vi "Add Error to Display.vi"(8 "error in (no error)":errorcluster, 9 "Update Listbox":bool=TRUE, 10 "error to display":T1 {"Time Stamp" format="%<%x %.3X>T"}, 11 "Error Manager in":refnum<class "Error Manager.lvclass">) -> (0 "error out":errorcluster, 3 "Error Manager out":refnum<class "Error Manager.lvclass">)   [LabVIEW 2026, in "TALOS.lvlib" / "Error Manager.lvlib" / "Error Manager.lvclass"]
uses:
  Error Manager.lvclass
  C:/LabVIEW Code/TALOS/talos/Father of all uServices/Father of all uServices/Father of all uServices.lvclass
  Error Info.ctl
  Error Manager.lvclass/Error Manager.ctl
  Father of all uServices/Father of all uServices/Father of all uServices.lvclass/Father of all uServices.ctl
  Ancestor/Ancestor/Ancestor.lvclass/Ancestor.ctl
  Common GUI v3/Common GUI v3/Error Listbox Msg.ctl
  Common GUI v3/Common GUI v3/Error Listbox Msg Action.ctl
  Guardian/Guardian/Requests.ctl
  Guardian/Guardian Messages/Requests from uServices Msg/Requests from uServices Msg.lvclass/Requests from uServices Msg.ctl
  Support VIs/Substitute Error.vi
  Guardian/Guardian Messages/Requests from uServices Msg/Send Requests from uServices.vi
  Support VIs/Generate Error.vi
  FGV/Error Memory/Get Error Description.vi
  Support VIs/Get PC name.vi
  Ancestor/Ancestor/Read ID.vi
  Support VIs/Get Class Name.vi
  <vilib>/Utility/error.llb/Clear Errors.vi
  FGV/Error Memory/Error Memory Core.vi
  <vilib>/AdvancedString/Delimited String to 1D String Array.vi
  <vilib>/AdvancedString/Delimited String to 1D String Array (string).vi
  Support VIs/Circus Root Path.vi
  FGV/Error Memory/Error Crt Lvl checker.vi
  FGV/Error Memory/Error Memory Core.vi/40c8088d-b597-4017-91af-faa98e00292e.vi
  FGV/Error Memory/Error Memory Core.vi/d4a3ab98-063c-4e44-b43d-fbdcfe6c2be2.vi
  Father of all uServices/Father of all uServices/Father of all uServices.lvclass
  C:/LabVIEW Code/TALOS/builds/Actor Framework PPL/Actor Framework.lvlibp/1abvi3w/vi.lib/ActorFramework/Actor/Actor.lvclass
  Support VIs/Global Memory.vi
  <vilib>/Utility/LVClass/Get LV Class Name.vi
  Support VIs/Is in Packed Library.vi
  Support VIs/TALOS Root path.vi
  Support VIs/Read CSV worksheet.vi
  Support VIs/Global Constants.vi
  <vilib>/Utility/error.llb/General Error Handler.vi
  Support VIs/Error Log.vi
  builds/Actor Framework PPL/Actor Framework.lvlibp/1abvi3w/vi.lib/ActorFramework/Actor/Read Caller Enqueuer.vi
  builds/Actor Framework PPL/Actor Framework.lvlibp/1abvi3w/vi.lib/ActorFramework/Message Enqueuer/Enqueue.vi
  Ancestor/Ancestor/Ancestor.lvclass
  <vilib>/Comparison/Equal/Equal Functor/Equal Functor.lvclass
  Guardian/Guardian Messages/Requests from uServices Msg/Requests from uServices Msg.lvclass
  Guardian/Guardian/Guardian.lvclass
  Common GUI v3/Common GUI v3/Common GUI v3.lvclass
  TALOS.lvlib
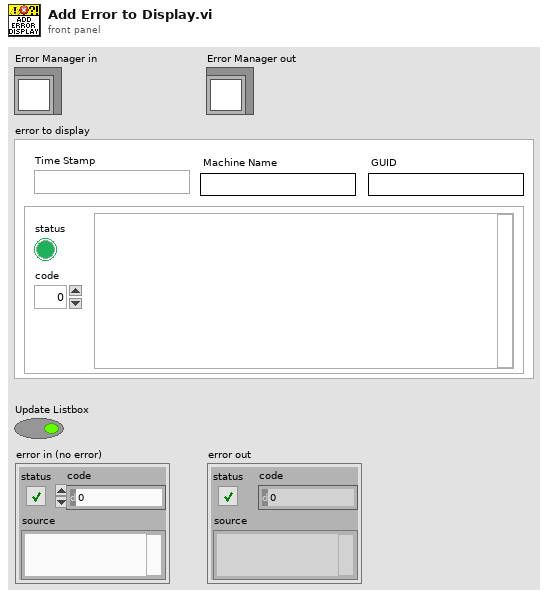
[diagram p1: front panel]
types:
  T1 = typedef "TALOS.lvlib/Error Manager.lvlib/Error Manager.lvclass/Error Info.ctl" = cluster{"error out":errorcluster, "Time Stamp":timestamp, "Machine Name":string, "GUID":string}
  T2 = typedef "TALOS.lvlib/Guardian.lvlib/Guardian.lvclass/Requests.ctl" = enum16{"Ready to Launch", "Start RUN", "Stop RUN", "Update DAQ Params", "Update Error Listbox", "Update Run Status", "Update Kasli Log", "Run Stopped with Errors", "Switch uS View", "Dismiss All Errors"}
  T3 = typedef "TALOS.lvlib/Common GUI v3.lvlib/Common GUI v3.lvclass/Error Listbox Msg Action.ctl" = enum16{"Add", "Remove", "Clear"}
  T4 = typedef "TALOS.lvlib/Common GUI v3.lvlib/Common GUI v3.lvclass/Error Listbox Msg.ctl" = cluster{"Action":T3, "Error Info":T1}
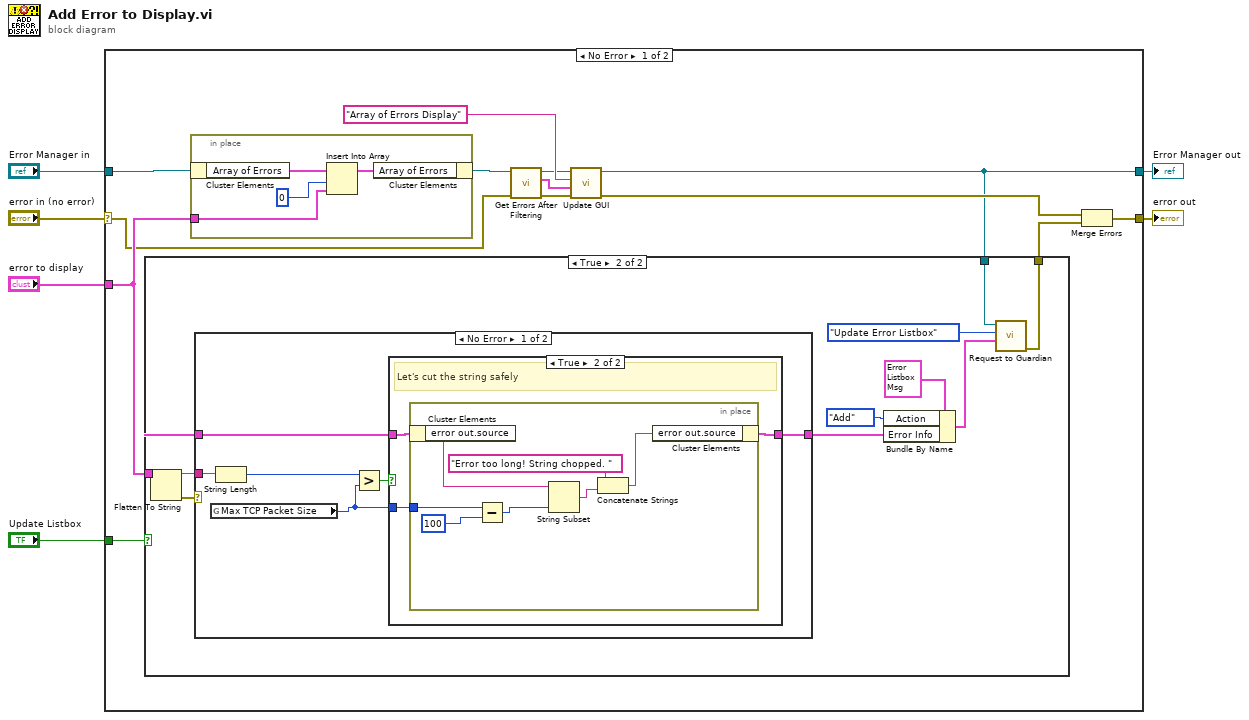
[diagram p0: block diagram]
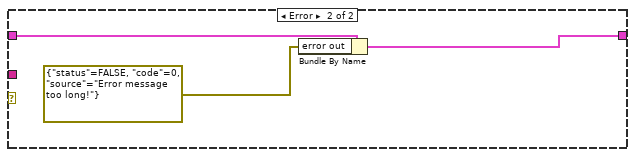
[diagram p4: hidden frame]
diagram:
  n1 = case shown="No Error" "error in (no error)" {
    selector: "error in (no error)" -> [w9 w55]
    tunnel: [w8 w54] -> w6
    tunnel: "error to display" -> [w14 _]
    tunnel: "Error Manager in" -> [w16 w54]
    tunnel: [w19 w55] -> w2
    tunnel: "Update Listbox" -> [w7 _]
    frame No Error {
      n2 = in-place {
        in-place-border: w14 -> [w51]
        n3 = in-place-cluster #1(w16) -> ("Array of Errors"=w53:T1[])
        n4 = Insert Into Array(array=w53, index=0, new element=w51) -> (w52:T1[])
        n5 = in-place-cluster #1("Array of Errors"=w52) -> (w15:refnum<class "Error Manager.lvclass">)
      }
      n6 = call-dynamic "Get Errors After Filtering.vi"("error in (no error)"=w9, "Error Manager in"=w15) -> ("error out"=w10:errorcluster, "Array of Errors"=w11:T1[], "Error Manager out"=w12:refnum<class "Error Manager.lvclass">)  [unwired: 7 in]
      n7 = call "Update GUI.vi"("error in (no error)"=w10, "Data"=w11, "GUI Item Name"="Array of Errors Display" ("FP Item Name"), "uService Template in"=w12) -> ("error out"=w17:errorcluster, "uService Template out"=w8:refnum<class "Error Manager.lvclass">)  [unwired: 6 in]
      n8 = case shown="True" w7 {
        tunnel: [_ w28] -> w18
        tunnel: w14 -> [_ w24]
        tunnel: w8 -> [_ w21]
        frame False {
        }
        frame True {
          n9 = Flatten To String(anything=w24) -> (data string=w27:string, error out=w26:errorcluster)  [unwired: 3 in, 1 out]
          n10 = case shown="No Error" w26 {
            tunnel: w27 -> [w35 _]
            tunnel: w24 -> [w33 w49]
            tunnel: [w31 w48] -> w25
            frame No Error {
              n11 = global read "Global Constants.vi" "Max TCP Packet Size"() -> (w30:i32)
              n12 = String Length(string=w35) -> (length=w34:i32)
              n13 = Greater?(x=w34, y=w30) -> (0:w32:bool)
              n14 = case shown="True" w32 {
                tunnel: w33 -> [w36 w39]
                tunnel: [w36 w38] -> w31
                tunnel: w30 -> [_ w37]
                frame False {
                  # "Length OK, send it."
                }
                frame True {
                  # "Let's cut the string safely"
                  n15 = in-place {
                    in-place-border: w37 -> [w45]
                    n16 = in-place-cluster #2(w39) -> ("error out.source"=w46:string)
                    n17 = Subtract(x=w45, y=u16 100) -> (x-y=w43:i32)
                    n18 = String Subset(string=w46, length (rest)=w43) -> (substring=w42:string)  [unwired: 1 in]
                    n19 = Concatenate Strings("Error too long! String chopped. " ("source"), w42) -> (w40:string)
                    n20 = in-place-cluster #2("error out.source"=w40) -> (w38:T1)
                  }
                }
              }
            }
            frame Error {
              n21 = Bundle By Name(cluster=w49, "error out"=errorcluster {"status"=FALSE, "code"=0, "source"="Error message too long!"}) -> (w48:T1)
            }
          }
          n22 = Bundle By Name(cluster=T4 {"Action"=enum."Add", "Error Info"={"error out"={"status"=FALSE, "code"=0, "source"=""}, "Time Stamp"=timestamp(0 s since 1904-01-01), "Machine Name"="", "GUID"=""}} ("Error Listbox Msg"), "Action"=Error_Listbox_Msg_Action."Add", "Error Info"=w25) -> (w22:T4)
          n23 = call "Request to Guardian.vi"("Data"=w22, "Requests"=Requests."Update Error Listbox", "Father of all uServices in"=w21) -> ("error out"=w28:errorcluster)  [unwired: 7 in, 1 out]
        }
      }
      n24 = Merge Errors(w17, w18) -> (w19:errorcluster)
    }
    frame Error {
    }
  }
  "Error Manager out" <- w6
  "error out" <- w2
